vi "Get Data.vi"(8 "error in":errorcluster, 11 "tCRD in":refnum<class "tCRD.lvclass">) -> (0 "error out":errorcluster, 3 "tCRD out":refnum<class "tCRD.lvclass">)   [LabVIEW 2015, in "tCRD.lvclass"]
doc: "Retrieve the data from the given cards. Set the <B>goodData</B> flag to True and log any errors that will be handled down the line. If there is an error associated with the collection of the data, the <B>goodData</B> flag will be set to false when the logged errors are handled.\nThe ringdown traces recorded in the <B>HF AI</B> task are divided up into a m x n matrix where:\n * m = YAG pulse rate\n * n = YAG duty cycle * HF AI Sampling Rate / YAG Pulse Rate"
uses:
  tCRD.lvclass
  Reusable/Instrument/Instrument.lvclass
  Reusable/Instrument/state.ctl
  tFPGA Ref.ctl
  <vilib>/rvi/interface/nirviReadWriteControl/nirviReadWriteControl.xnode
  Reusable/CRDS/Data/Cell/CRDS Cell Data.lvclass
  Reusable/CRDS/Cell/CRDS Cell.lvclass
  Reusable/CRDS/Data/Main/CRDS Data.lvclass
  Devices/Alicat/Session Based/Data/Alicat Data.lvclass
  Data/tCRD Data.lvclass
  Devices/Alicat/Session Based/Alicat Device.lvclass
  FPGA Bitfiles/FPGAServerwLRS.lvbitx
  NiFpgaLv.dll
  <vilib>/Utility/error.llb/Error Cluster From Error Code.vi
  <vilib>/rvi/errors/niLvFpgaAdjustHostInterfaceError.vi
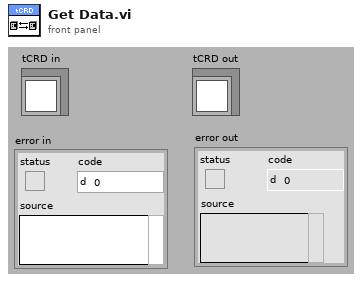
[diagram p1: front panel]
types:
  T1 = typedef "Instrument.lvclass/state.ctl" = enum8{"Configure", "Acquire", "Wait", "Quit", "Handle Error", "NOOP"}
  T2 = typedef "tCRD.lvclass/tFPGA Ref.ctl" = refnum<k20>
  T3 = cluster{"RH":fxp<+,16,8>, "T":fxp<+/-,16,8>, "Velocity":fxp<+/-,16,8>}
  T4 = typedef "calData.ctl" = cluster{"rhDilFac":sgl, "Q":sgl, "Tmean":sgl, "extDilFac":sgl, "rhCell":sgl, "P":sgl, "T":sgl}
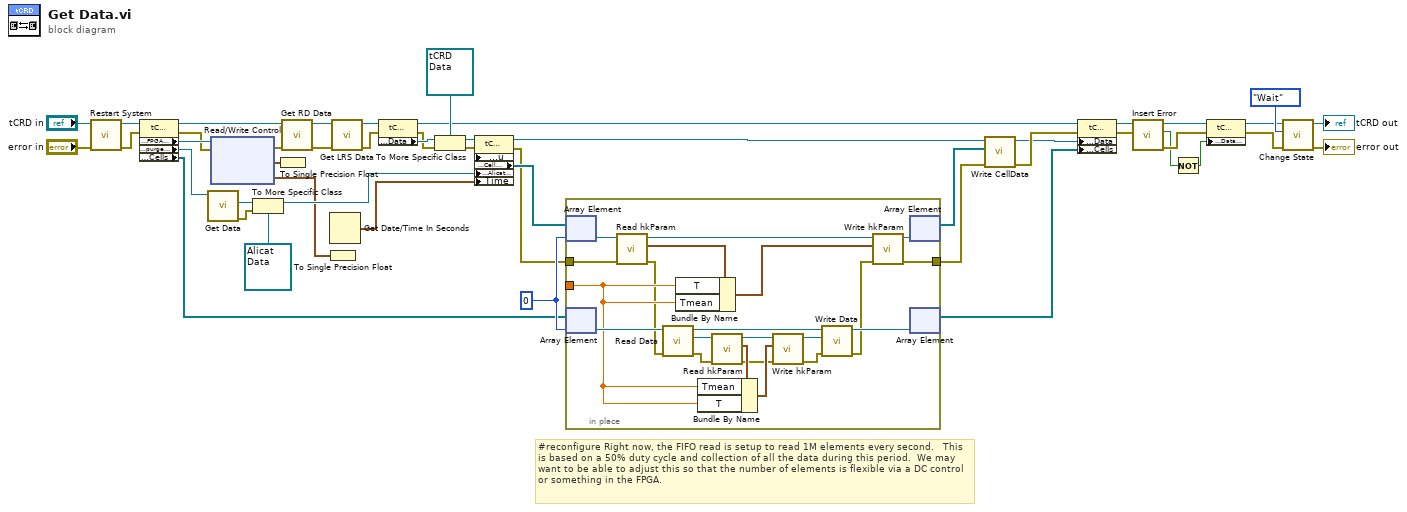
[diagram p0: block diagram]
diagram:
  w37 = 0
  # "#reconfigure Right now, the FIFO read is setup to read 1M elements every second.   This is based on a 50% duty cycle and collection of all the data during this period.  We may want to be able to adjust this so that the number of elements is flexible via a DC control or something in the FPGA."
  n1 = call "Restart System.vi"("error in"="error in", "tCRD in"="tCRD in") -> ("error out"=w31:errorcluster, "tCRD out"=w30:refnum<class "tCRD.lvclass">)  [unwired: 8 in]
  n2 = property class="tCRD"(reference=w30, error in=w31) -> (reference out=w18:refnum<class "tCRD.lvclass">, error out=w35:errorcluster, "Accessors:FPGA Ref"=w36:T2, "Accessors:purgeFlow"=w24:refnum<class "Alicat Device.lvclass">, "Data Access:Cells"=w3:refnum<class "CRDS Cell.lvclass">[])
  n3 = call-dynamic "Get Data.vi"("Cfg Dev in"=w24) -> ("error out"=w21:errorcluster, "DataOut"=w23:refnum<class "Data.lvclass">)  [unwired: 8 in, 1 out]
  n4 = xnode "Read/Write Control"("FPGA VI Reference In"=w36, "error in"=w35) -> ("error out"=w34:errorcluster, "LF Data"=w38:T3, "Rotronic"=w1:cluster{"RH":fxp<+,16,8>, "T":fxp<+/-,16,8>})  [unwired: 1 out]
  n5 = To More Specific Class(target class=refnum<class "Alicat Data.lvclass"> refnum ("Alicat Data"), reference=w23, error in=w21) -> (specific class reference=w19:refnum<class "Alicat Data.lvclass">)  [unwired: 1 out]
  n6 = To Single Precision Float(number=w38) -> ()  [unwired: 1 out]
  n7 = call "Get RD Data.vi"("error in"=w34, "tCRD in"=w18) -> ("error out"=w5:errorcluster, "tCRD out"=w17:refnum<class "tCRD.lvclass">)  [unwired: 8 in]
  n8 = To Single Precision Float(number=w1) -> ()  [unwired: 1 out]
  n9 = Get Date/Time In Seconds() -> (seconds since 1Jan1904=w2:timestamp)
  n10 = call "Get LRS Data.vi"("error in"=w5, "tCRD in"=w17) -> ("error out"=w9:errorcluster, "tCRD out"=w16:refnum<class "tCRD.lvclass">)  [unwired: 8 in]
  n11 = property class="tCRD"(reference=w16, error in=w9) -> (reference out=w12:refnum<class "tCRD.lvclass">, error out=w8:errorcluster, "Data Access:Data"=w14:refnum<class "CRDS Data.lvclass">)
  n12 = To More Specific Class(target class=refnum<class "tCRD Data.lvclass"> refnum ("tCRD Data"), reference=w14, error in=w8) -> (specific class reference=w11:refnum<class "tCRD Data.lvclass">, error out=w10:errorcluster)
  n13 = property class="tCRD Data" props=["Accessors:u", "Data Access:Cell Data", "Accessors:Alicat Data", "Time"](reference=w11, error in=w10, "Accessors:Alicat Data"=w19, "Time"=w2) -> (reference out=w15:refnum<class "tCRD Data.lvclass">, error out=w4:errorcluster, "Data Access:Cell Data"=w20:refnum<class "CRDS Cell Data.lvclass">[])  [unwired: 1 in]
  n14 = in-place {
    in-place-border: _ -> [w53]
    in-place-border: w4 -> [w67]
    in-place-border: [w63] -> w28
    n15 = in-place-array #1(w20, w37) -> (w68:refnum<class "CRDS Cell Data.lvclass">)
    n16 = in-place-array #2(w3, w37) -> (w61:refnum<class "CRDS Cell.lvclass">)
    n17 = call "Read hkParam.vi"("error in"=w67, "CRDS Cell Data in"=w68) -> ("error out"=w48:errorcluster, "hkParam"=w66:T4, "CRDS Cell Data out"=w65:refnum<class "CRDS Cell Data.lvclass">)  [unwired: 7 in]
    n18 = call "Read Data.vi"("error in"=w48, "CRDS Cell in"=w61) -> ("error out"=w51:errorcluster, "CRDS Cell"=w59:refnum<class "CRDS Cell Data.lvclass">, "CRDS Cell out"=w60:refnum<class "CRDS Cell.lvclass">)  [unwired: 7 in]
    n19 = Bundle By Name(cluster=w66, "T"=w53, "Tmean"=w53) -> (w62:T4)
    n20 = call "Read hkParam.vi"("error in"=w51, "CRDS Cell Data in"=w59) -> ("error out"=w50:errorcluster, "hkParam"=w56:T4, "CRDS Cell Data out"=w57:refnum<class "CRDS Cell Data.lvclass">)  [unwired: 7 in]
    n21 = Bundle By Name(cluster=w56, "Tmean"=w53, "T"=w53) -> (w55:T4)
    n22 = call "Write hkParam.vi"("error in (no error)"=w50, "hkParam"=w55, "CRDS Cell Data in"=w57) -> ("error out"=w49:errorcluster, "CRDS Cell Data out"=w54:refnum<class "CRDS Cell Data.lvclass">)  [unwired: 7 in]
    n23 = call "Write Data.vi"("error in"=w49, "CRDS Cell"=w54, "CRDS Cell in"=w60) -> ("error out"=w52:errorcluster, "CRDS Cell out"=w58:refnum<class "CRDS Cell.lvclass">)  [unwired: 7 in]
    n24 = call "Write hkParam.vi"("error in (no error)"=w52, "hkParam"=w62, "CRDS Cell Data in"=w65) -> ("error out"=w63:errorcluster, "CRDS Cell Data out"=w64:refnum<class "CRDS Cell Data.lvclass">)  [unwired: 7 in]
    n25 = in-place-array #1(w64) -> (w29:refnum<class "CRDS Cell Data.lvclass">[])  [unwired: 1 out]
    n26 = in-place-array #2(w58) -> (w25:refnum<class "CRDS Cell.lvclass">[])  [unwired: 1 out]
  }
  n27 = call "Write CellData.vi"("error in"=w28, "CellData"=w29, "CRDS Data in"=w15) -> ("error out"=w27:errorcluster, "CRDS Data out"=w26:refnum<class "tCRD Data.lvclass">)  [unwired: 7 in]
  n28 = property class="tCRD"(reference=w12, error in=w27, "Data Access:Data"=w26, "Data Access:Cells"=w25) -> (reference out=w7:refnum<class "tCRD.lvclass">, error out=w6:errorcluster)
  n29 = call "Insert Error.vi"("err"=w6, "Instrument in"=w7) -> ("error out"=w43:errorcluster, "error?"=w40:bool, "Instrument out"=w44:refnum<class "tCRD.lvclass">)  [unwired: 7 in]
  n30 = Not(x=w40) -> (.not. x?=w39:bool)
  n31 = property class="tCRD"(reference=w44, error in=w43, "Data Access:Data Ready?"=w39) -> (reference out=w42:refnum<class "tCRD.lvclass">, error out=w41:errorcluster)
  n32 = call "Change State.vi"("error in"=w41, "instr state"=state."Wait", "Instrument in"=w42) -> ("error out"=→"error out":errorcluster, "Instrument out"=→"tCRD out":refnum<class "tCRD.lvclass">)  [unwired: 7 in]
